vi "FV_Parameter.vi"(8 "error in (no error)":errorcluster, 11 "Ref in":T3={"MS SQL Connection"=refnum, "UDL File"=path "", "Time"="", "DCODE"="", "WIP+1"=0, "MC No?"=0, "POKAYOKE?"=FALSE, "Expected Result"="", "Result [Status]"="", "Clock"=0.0, "RFID"="", "WIP Queue"=refnum, "TS Parameter"={"ProfitCenterCode"="", "LineCode"="", "WorkOrderNumber"="", "Model"="", "Model_with_Prefix"="", "VendorCode"="", "SetParameterDateCode"="", "PokaYoke"=0, "Target"=1, "Live_DateCode"="", "CustomerPartNumber"="", "Hand"="", "sBarcode"=FALSE, "FCA"=0, "Ent_Stamp"=timestamp(0 s since 1904-01-01), "STS_CD"=0.0}, "Data_Queue"=[], "RFID Serial No."=""} {"TS Parameter"."FCA" format="%01d"; "TS Parameter"."Target" min=1 max=100000; "TS Parameter"."PokaYoke" min=0 max=1}) -> (0 "error out":errorcluster)   [LabVIEW 2020]
uses:
  Controls/TD SQL.ctl
  <vilib>/addons/database/Connection.llb/Conn ObjectReference.ctl
  Controls/WIP_State.ctl
  Controls/TS_Parameter.ctl
  Controls/FV_Operator.ctl
  <vilib>/Utility/miscctls.llb/LVPointTypeDef.ctl
  <vilib>/Utility/miscctls.llb/LVRowAndColumnUnsignedTypeDef.ctl
  <userlib>/_OpenG.lib/array/array.llb/Delete Elements from 1D Array (String)__ogtk.vi
  <vilib>/addons/database/NI_Database_API.lvlib
panel:
  in  "Exit":bool
  in  "Save wip":bool
  out "size(s)":i32
  in  "Add":bool
  in  "Remove":bool
  in  "Checking Tags":i32(listbox)
  in  "Avaliable Tags":i32(listbox)
  in  "FV_Check":T2 {"Tags" items=["PROFITCENTRE", "DTS_SCAN", "DTS_PASS", "DCODE", "SERIAL_NO", "BLEED_PORT_CNTY", "INLET_PORT_CNTY", "BLEED_TEST_TIME", "CLEANING_VAC", "CT", "STATUS", "FCS", "FCA", "ROUTING", "MODELNO", "WORKORDER", "CELLNO", "PROFITCENTRE", "MACHINECODE", "OPERATIONCODE", "RESERVED_1", "RESERVED_2", "RESERVED_3", "RESERVED_4", "RESERVED_5"]}
  out "Tags":string[](array[string])
  in  "Machine No":u16(ring) items=["OP20A", "OP20A", "OP20A", "OP20A"]
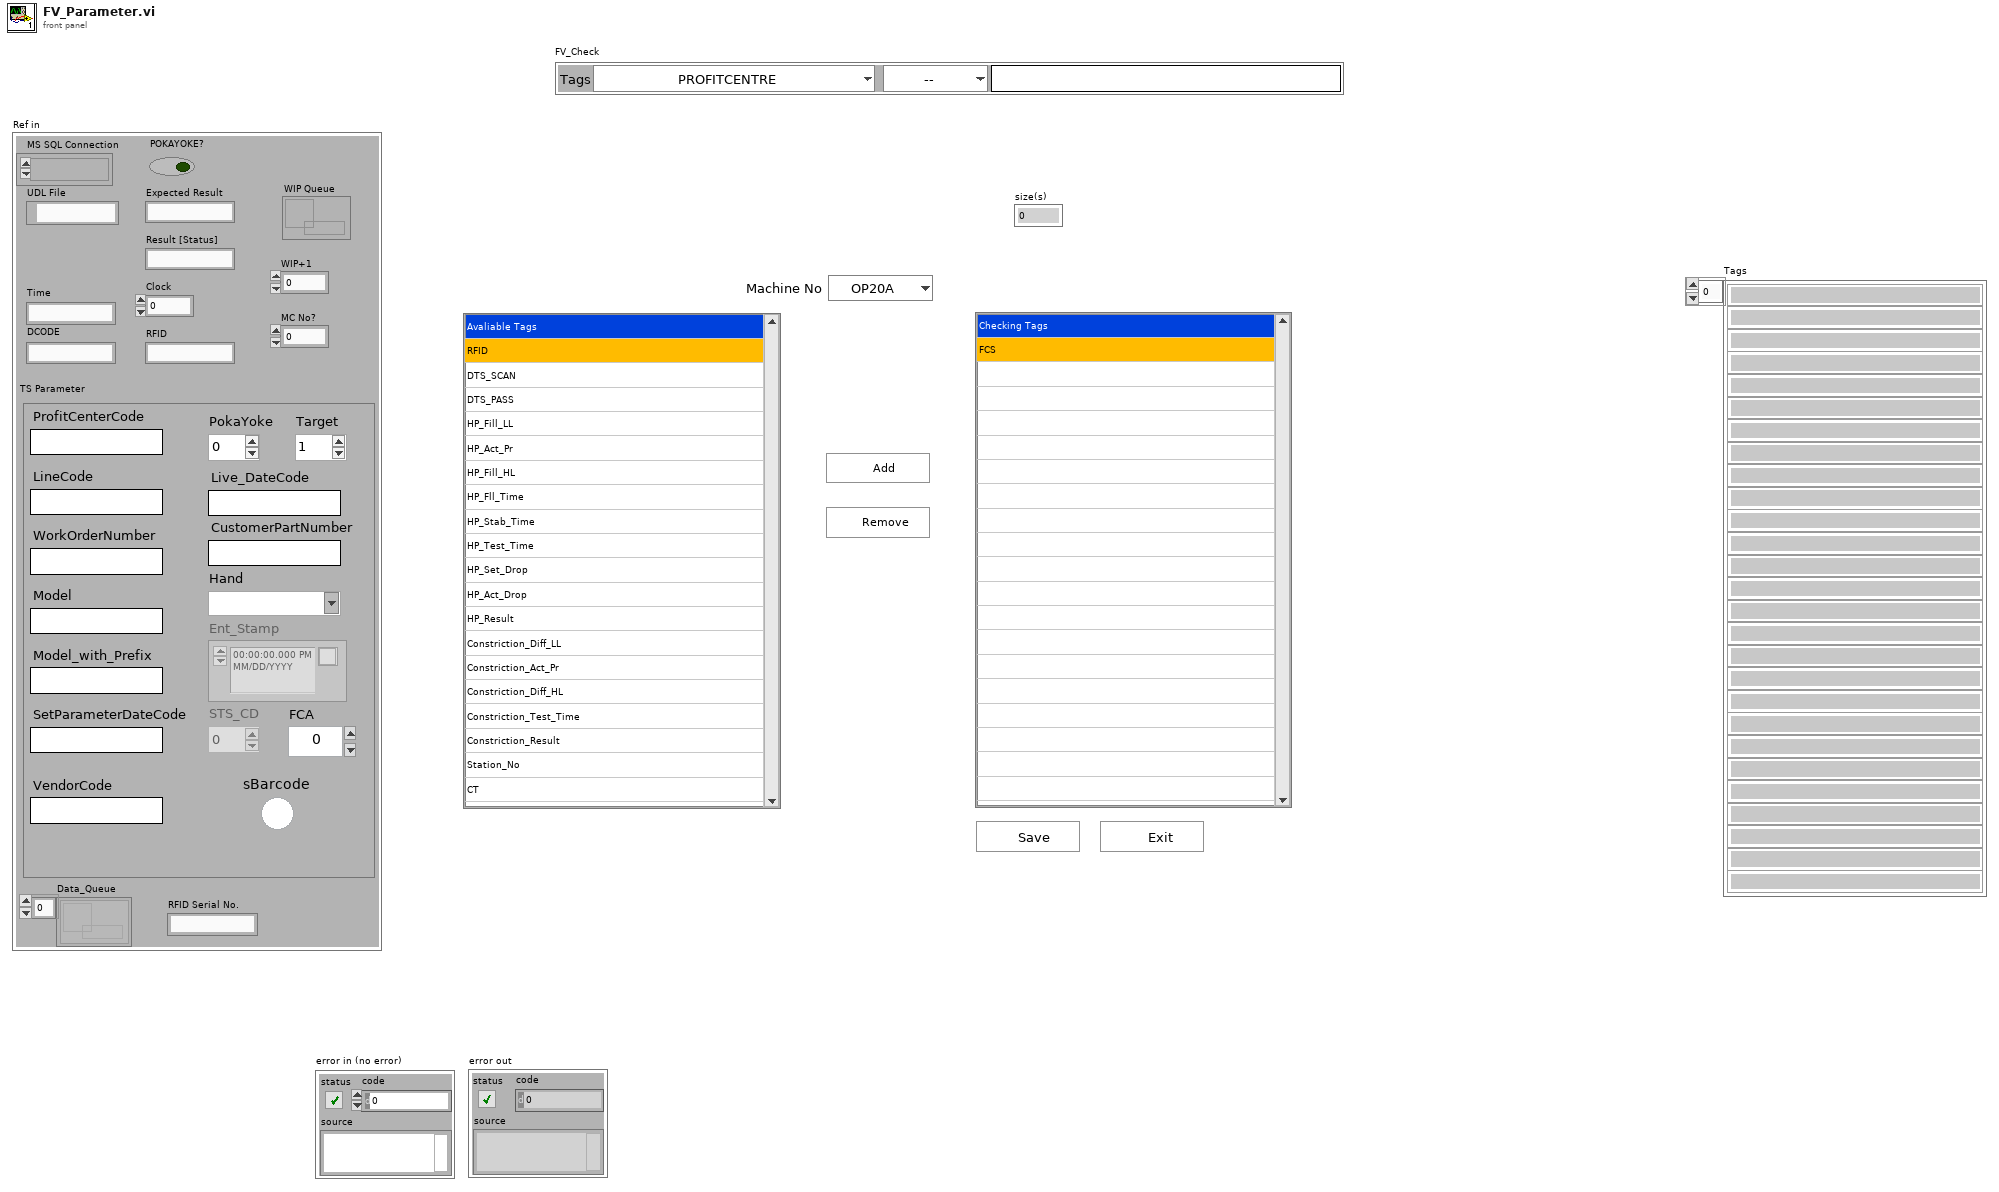
[diagram p1: front panel]
types:
  T1 = typedef "FV_Operator.ctl" = enum16{"--", "<", ">", "=", "Limits"}
  T2 = cluster{"Tags":u16, "Operator":T1, "Field":string}
  T3 = typedef "TD SQL.ctl" = cluster{"MS SQL Connection":T4, "UDL File":path, "Time":string, "DCODE":string, "WIP+1":i64, "MC No?":i32, "POKAYOKE?":bool, "Expected Result":string, "Result [Status]":string, "Clock":dbl, "RFID":string, "WIP Queue":refnum<queue>, "TS Parameter":T5, "Data_Queue":refnum<queue>[], "RFID Serial No.":string}
  T4 = typedef "NI_Database_API.lvlib/Conn ObjectReference.ctl" = refnum<k1>
  T5 = typedef "TS_Parameter.ctl" = cluster{"ProfitCenterCode":string, "LineCode":string, "WorkOrderNumber":string, "Model":string, "Model_with_Prefix":string, "VendorCode":string, "SetParameterDateCode":string, "PokaYoke":i32, "Target":i32, "Live_DateCode":string, "CustomerPartNumber":string, "Hand":string, "sBarcode":bool, "FCA":i32, "Ent_Stamp":timestamp, "STS_CD":dbl}
  T6 = typedef "LVPointTypeDef.ctl" = cluster{"Horizontal":i16, "Vertical":i16}
  T7 = enum8{"Enabled", "Disabled", "Disabled and Grayed Out"}
  T8 = typedef "LVRowAndColumnUnsignedTypeDef.ctl" = cluster{"Row":u32, "Column":u32}
  T9 = cluster{"data name":string, "drag data":variant}[]
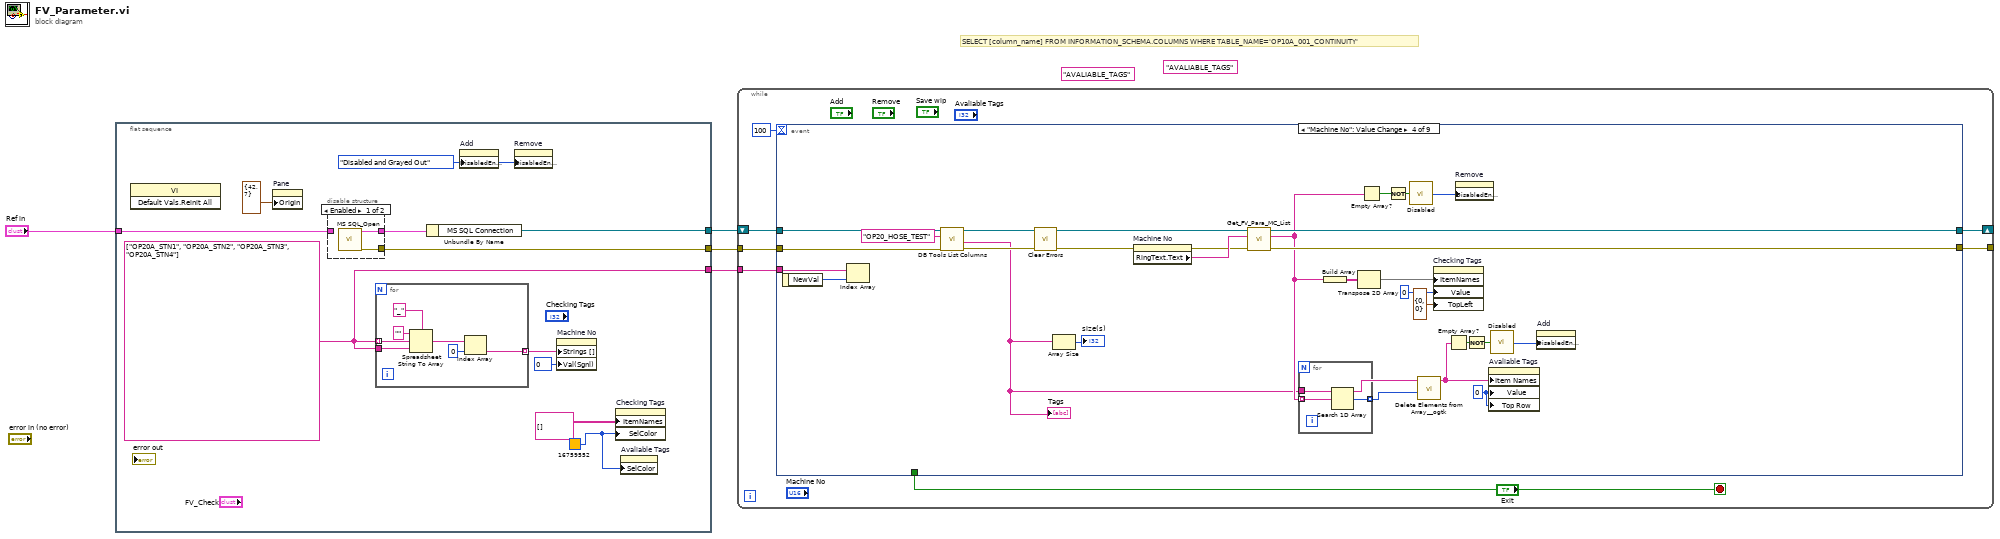
[diagram p0: block diagram]
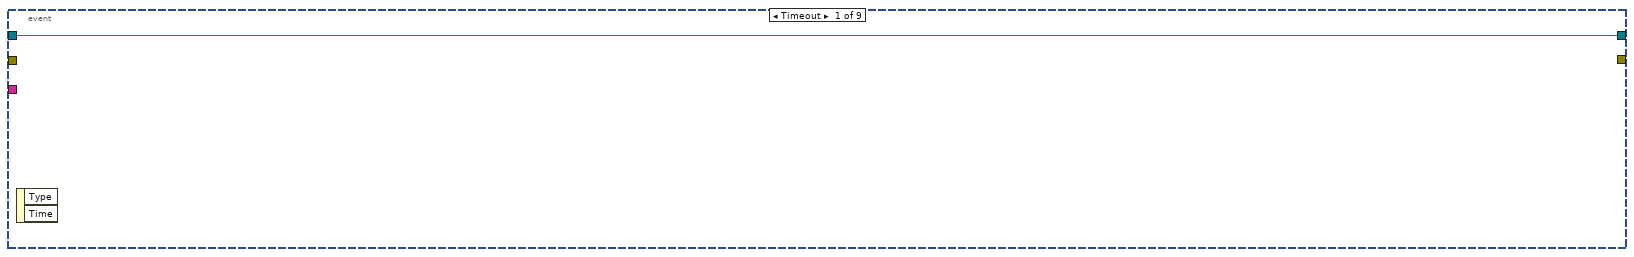
[diagram p3: hidden frame]
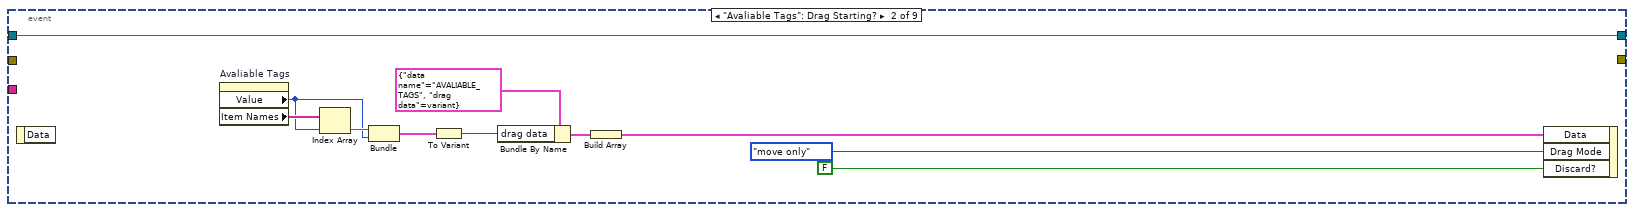
[diagram p4: hidden frame]
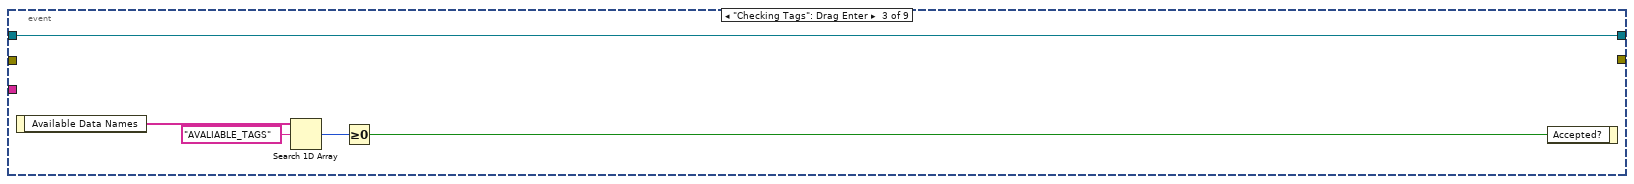
[diagram p5: hidden frame]
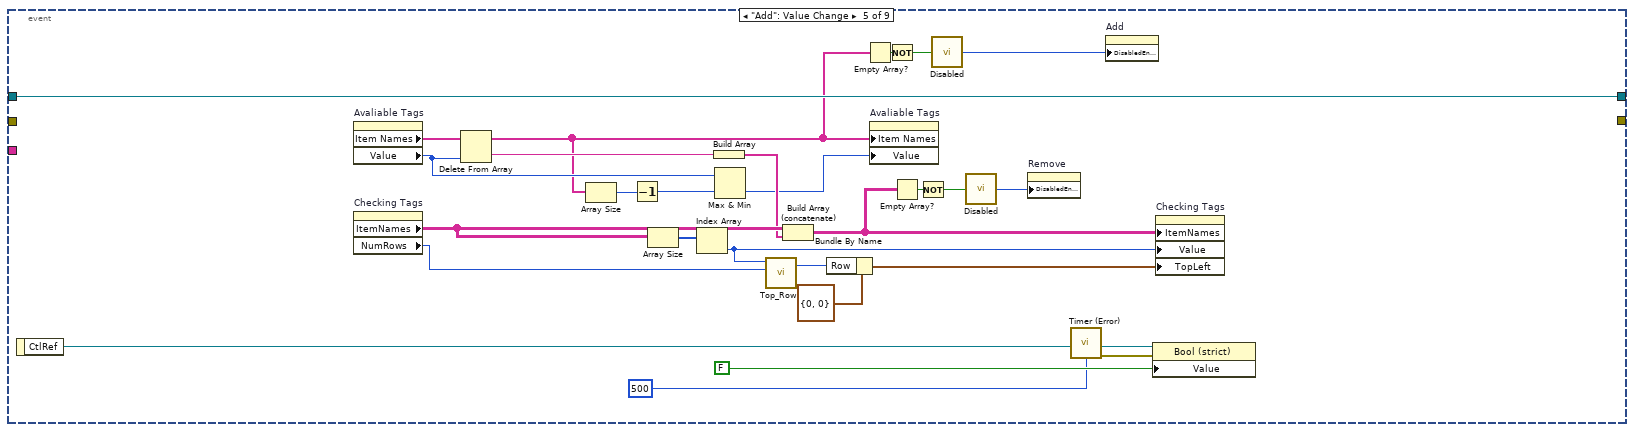
[diagram p6: hidden frame]
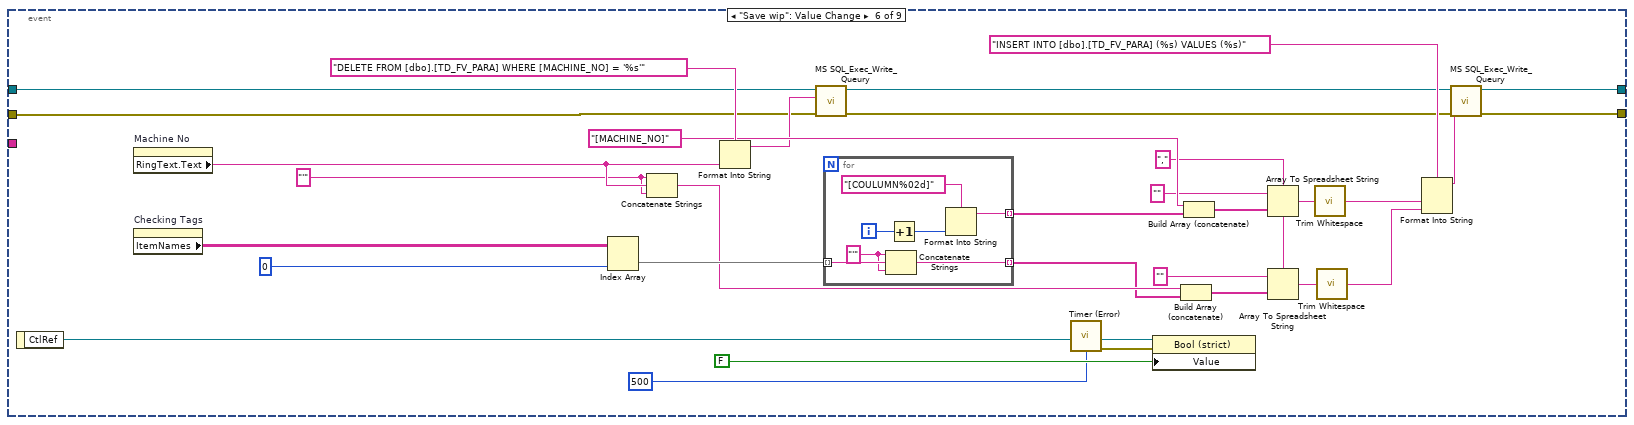
[diagram p7: hidden frame]
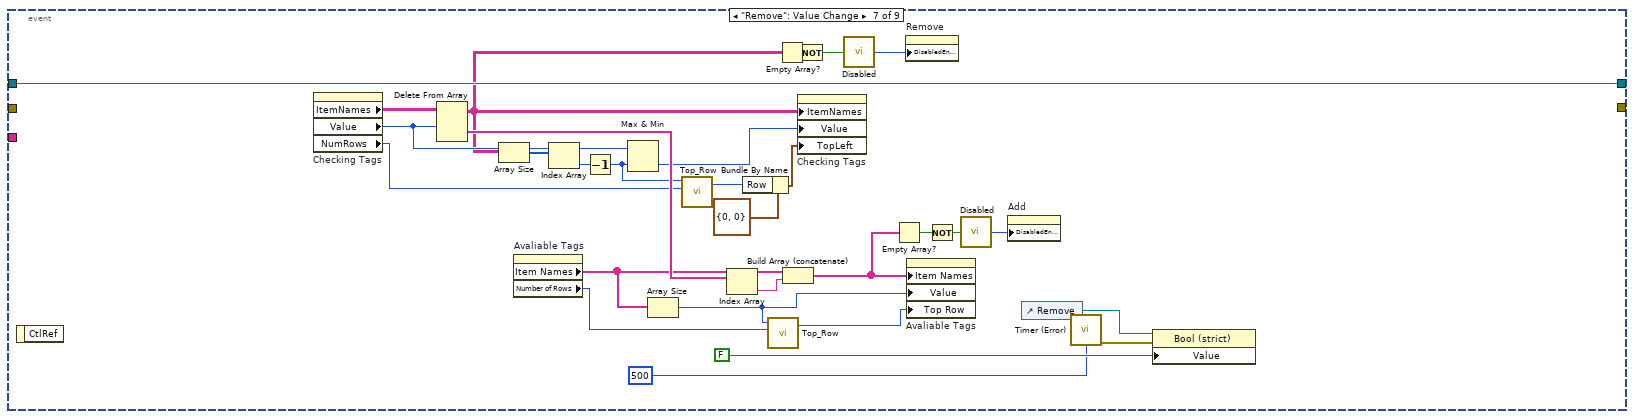
[diagram p8: hidden frame]
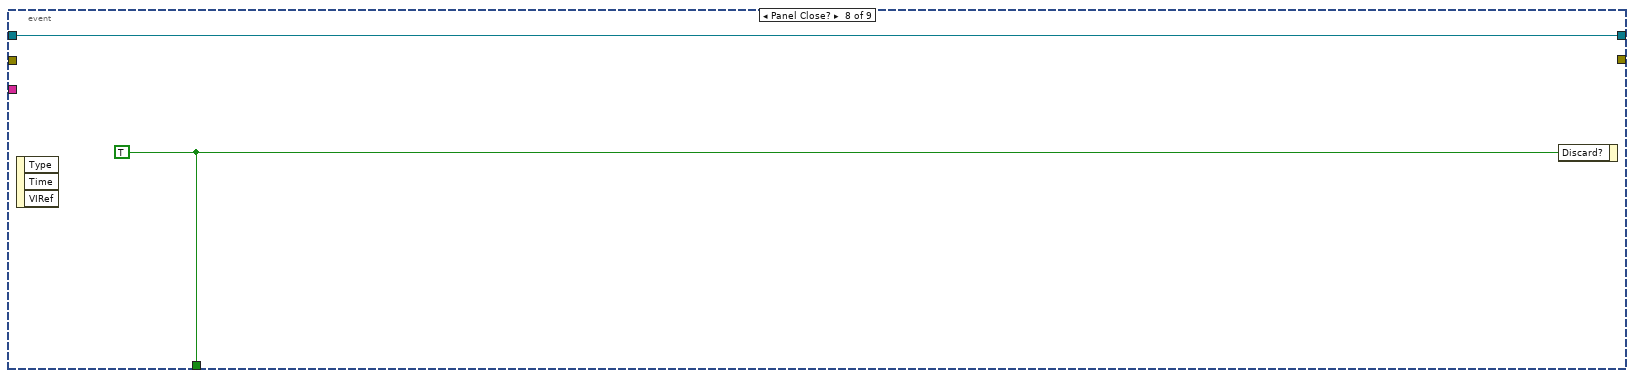
[diagram p9: hidden frame]
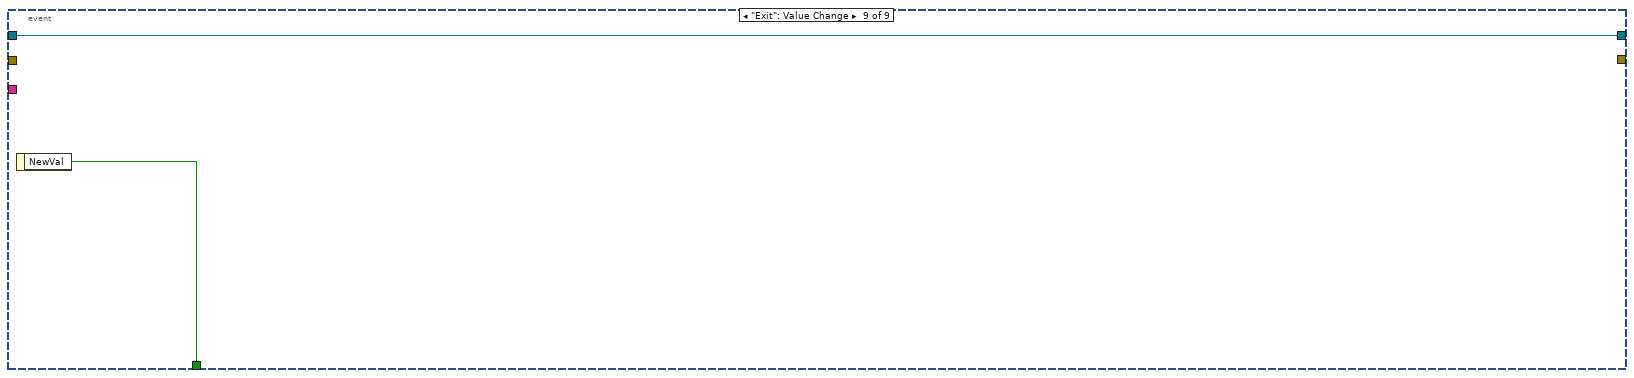
[diagram p10: hidden frame]
diagram:
  (unwired) "AVALIABLE_TAGS" ("data name")
  (unwired) "AVALIABLE_TAGS" ("data name")
  # "SELECT [column_name] FROM INFORMATION_SCHEMA.COLUMNS WHERE TABLE_NAME='OP10A_001_CONTINUITY'"
  n1 = flat-sequence {
    tunnel: "Ref in" -> [w14]
    tunnel: [w11] -> w1
    tunnel: [w10] -> w3
    tunnel: [w9] -> w2
    frame #0 {
      w6 = T7."Disabled and Grayed Out" ("Disabled")
      w7 = u32 16759552 ("Selection Color")
      w12 = u16 0 items=[""] ("Machine No")
      w10 = string[] ["OP20A_STN1", "OP20A_STN2", "OP20A_STN3", "OP20A_STN4"] ("tables 2")
      n2 = invoke class="VI" method="Default Vals.Reinit All"() -> ()  [unwired: 3 in, 3 out]
      n3 = property on="Pane" class="Pane"("Origin"=T6 {"Horizontal"=42, "Vertical"=7}) -> ()  [unwired: 2 in, 2 out]
      n4 = disable-structure shown="Enabled" {
        disable-tunnel: [w24 w25] -> w15
        disable-tunnel: w14 -> [_ w25]
        disable-tunnel: [w23 _] -> w9
        frame Enabled {
          n5 = call "MS SQL_Open.vi"() -> ("error out"=w23:errorcluster, "Ref Out"=w24:T3)  [unwired: 9 in, 1 out]
        }
        frame Disabled {
        }
      }
      n6 = for {
        tunnel: w10 -> [w18] mode=indexing
        tunnel: w10 -> [w17]
        tunnel: [w16] -> w13 mode=indexing
        n7 = Spreadsheet String To Array(delimiter (Tab)="_", format string="", spreadsheet string=w18, array type (2D Dbl)=w17) -> (array=w20:string[])
        n8 = Index Array(array=w20, index=0) -> (element=w16:string)
      }
      n9 = Unbundle By Name(w15) -> ("MS SQL Connection"=w11:T4)
      n10 = property on="Add" class="Bool (strict)"("DisabledEnum"=w6) -> ()  [unwired: 2 in, 2 out]
      n11 = property on="Remove" class="Bool (strict)"("DisabledEnum"=w6) -> ()  [unwired: 2 in, 2 out]
      n12 = property on="Machine No" class="Ring (strict)"("Strings []"=w13, "Val(Sgnl)"=w12) -> ()  [unwired: 2 in, 2 out]
      n13 = property on="Checking Tags" class="MCListbox (strict)"("ItemNames"=string[][] [] ("Item Names"), "SelColor"=w7) -> ()  [unwired: 2 in, 2 out]
      n14 = property on="Avaliable Tags" class="LstBox (strict)"("SelColor"=w7) -> ()  [unwired: 2 in, 2 out]
    }
  }
  n15 = while {
    tunnel: w3 -> [w31]
    tunnel: w2 -> [w30]
    tunnel: [w29] -> _
    shift-right: [w28] -> _
    shift-left: w1 -> [w27]
    stop <- w32 stop-if-true
    n16 = event shown="[3] \"Machine No\": Value Change" {
      selector: _ -> [_ _ _ _ _ _ _ _ _]
      dyn-events: _ -> [_ _ _ _ _ _ _ _ _]
      timeout: 100 -> [_ _ _ _ _ _ _ _ _]
      tunnel: [_ _ _ _ _ _ _ w177 w178] -> w32
      tunnel: w27 -> [w33 w44 w49 w66 w99 w115 w170 w176 w179]
      tunnel: w31 -> [_ _ _ w65 _ _ _ _ _]
      tunnel: w30 -> [_ _ _ w76 _ w113 _ _ _]
      tunnel: [_ _ _ w68 _ w109 _ _ _] -> w29
      tunnel: [w33 w44 w49 w69 w99 w108 w170 w176 w179] -> w28
      event Timeout {
        n17 = event-data() -> ()  [unwired: 1 in, 2 out]
      }
      event "Avaliable Tags": Drag Starting? {
        n18 = event-data() -> ()  [unwired: 1 in, 1 out]
        n19 = property on="Avaliable Tags" class="LstBox (strict)"() -> ("Value"=w39:i32, "Item Names"=w41:string[])  [unwired: 2 in, 2 out]
        n20 = Index Array(array=w41, index=w39) -> (element=w40:string)
        n21 = Bundle(w40, "Value"=w39) -> (w37:cluster{string, "Value":i32})  [unwired: 1 in]
        n22 = To Variant(anything=w37) -> (Variant=w34:variant)
        n23 = Bundle By Name(cluster=cluster{"data name":string, "drag data":variant} {"data name"="AVALIABLE_TAGS", "drag data"=variant}, "drag data"=w34) -> (w36:cluster{"data name":string, "drag data":variant})
        n24 = Build Array(w36) -> (w35:T9)
        n25 = event-data("Data"=w35, "Drag Mode"=enum32{"copy or move", "copy only", "move only"}."move only", "Discard?"=FALSE) -> ()  [unwired: 1 in, 1 out]
      }
      event "Checking Tags": Drag Enter {
        n26 = event-data() -> ("Available Data Names"=w47:string[])  [unwired: 1 in]
        n27 = Search 1D Array(1D array=w47, element="AVALIABLE_TAGS") -> (index of element=w48:i32)  [unwired: 1 in]
        n28 = Greater Or Equal To 0?(x=w48) -> (x >= 0?=w45:bool)
        n29 = event-data("Accepted?"=w45) -> ()  [unwired: 1 in, 1 out]
      }
      event "Machine No": Value Change {
        w56 = 0 ("Avaliable Tags")
        n30 = event-data() -> ("NewVal"=w77:u16)  [unwired: 1 in]
        n31 = Index Array(array=w65, index=w77) -> ()  [unwired: 1 out]
        n32 = call <vilib>:"DB Tools List Columns.vi"("error in (no error)"=w76, "table"="OP20_HOSE_TEST", "connection reference"=w66) -> ("error out"=w74:errorcluster, "columns"=w53:string[], "connection reference out"=w67:T4)  [unwired: 1 in, 1 out]
        "Tags" <- w53
        n33 = call <vilib>:"Clear Errors.vi"("error in (no error)"=w74) -> ("error out"=w52:errorcluster)  [unwired: 5 in, 1 out]
        n34 = Array Size(array=w53) -> (size(s)=→"size(s)":i32)
        n35 = property on="Machine No" class="Ring (strict)"(error in=w52) -> (error out=w51:errorcluster, "RingText.Text"=w72:string)  [unwired: 1 in, 1 out]
        n36 = call "Get_FV_Para_MC_List.vi"("error in (no error)"=w51, "Machine No."=w72, "Refnum in"=w67) -> ("error out"=w68:errorcluster, "Column"=w57:string[], "Refnum out"=w69:T4)  [unwired: 3 in, 3 out]
        n37 = for {
          tunnel: w53 -> [w80]
          tunnel: w57 -> [w79] mode=indexing
          tunnel: [w78] -> w70 mode=indexing
          n38 = Search 1D Array(1D array=w80, element=w79) -> (index of element=w78:i32)  [unwired: 1 in]
        }
        n39 = Build Array(w57) -> (w73:string[][])
        n40 = Transpose 2D Array(2D array=w73) -> (transposed array=w71:string[][])
        n41 = Empty Array?(array=w57) -> (empty?=w64:bool)
        n42 = Not(x=w64) -> (.not. x?=w59:bool)
        n43 = call <userlib>:"Disabled.vi"("Enable?"=w59) -> ("Disabled"=w63:T7)  [unwired: 14 in]
        n44 = call-poly <userlib>:"Delete Elements from Array__ogtk.vi"("indices"=w70, "array"=w53) -> ("array w/ subset deleted"=w60:string[])  [unwired: 8 in, 1 out]
        n45 = property on="Checking Tags" class="MCListbox (strict)"("ItemNames"=w71, "Value"=0 ("Checking Tags"), "TopLeft"=T8 {"Row"=0, "Column"=0} ("Top Left Visible Cell")) -> ()  [unwired: 2 in, 2 out]
        n46 = Empty Array?(array=w60) -> (empty?=w62:bool)
        n47 = property on="Remove" class="Bool (strict)"("DisabledEnum"=w63) -> ()  [unwired: 2 in, 2 out]
        n48 = Not(x=w62) -> (.not. x?=w58:bool)
        n49 = property on="Avaliable Tags" class="LstBox (strict)"("Item Names"=w60, "Value"=w56, "Top Row"=w56) -> ()  [unwired: 2 in, 2 out]
        n50 = call <userlib>:"Disabled.vi"("Enable?"=w58) -> ("Disabled"=w61:T7)  [unwired: 14 in]
        n51 = property on="Add" class="Bool (strict)"("DisabledEnum"=w61) -> ()  [unwired: 2 in, 2 out]
      }
      event "Add": Value Change {
        n52 = event-data() -> ("CtlRef"=w103:refnum<vi>)  [unwired: 1 in]
        n53 = property on="Avaliable Tags" class="LstBox (strict)"() -> ("Item Names"=w107:string[], "Value"=w97:i32)  [unwired: 2 in, 2 out]
        n54 = property on="Checking Tags" class="MCListbox (strict)"() -> ("ItemNames"=w105:string[][], "NumRows"=w82:u32)  [unwired: 2 in, 2 out]
        n55 = Delete From Array(array=w107, index=w97) -> (deleted portion=w106:string, array with subset deleted=w93:string[])  [unwired: 1 in]
        n56 = Array Size(array=w93) -> (size(s)=w96:i32)
        n57 = Decrement(x=w96) -> (x-1=w95:i32)
        n58 = Array Size(array=w105) -> (size(s)=w104:i32[])
        n59 = Index Array(array=w104) -> (element=w83:i32)  [unwired: 1 in]
        n60 = Build Array(w106) -> (w98:string[])
        n61 = Max & Min(x=w97, y=w95) -> (min(x,y)=w94:i32)  [unwired: 1 out]
        n62 = call "Top_Row.vi"("NumRows"=w82, "Step In"=w83) -> ("Step Out"=w81:i32)  [unwired: 3 in]
        n63 = Build Array (concatenate)(w105, w98) -> (w89:string[][])
        n64 = Bundle By Name(cluster=T8 {"Row"=0, "Column"=0} ("Top Left Visible Cell"), "Row"=w81) -> (w84:T8)
        n65 = Empty Array?(array=w93) -> (empty?=w92:bool)
        n66 = property on="Avaliable Tags" class="LstBox (strict)"("Item Names"=w93, "Value"=w94) -> ()  [unwired: 2 in, 2 out]
        n67 = Not(x=w92) -> (.not. x?=w87:bool)
        n68 = Empty Array?(array=w89) -> (empty?=w90:bool)
        n69 = Not(x=w90) -> (.not. x?=w86:bool)
        n70 = call <userlib>:"Disabled.vi"("Enable?"=w87) -> ("Disabled"=w91:T7)  [unwired: 14 in]
        n71 = call <userlib>:"Disabled.vi"("Enable?"=w86) -> ("Disabled"=w88:T7)  [unwired: 14 in]
        n72 = property on="Remove" class="Bool (strict)"("DisabledEnum"=w88) -> ()  [unwired: 2 in, 2 out]
        n73 = call <userlib>:"Timer (Error).vi"("milliseconds to wait"=u32 500) -> ("error out"=w100:errorcluster)  [unwired: 14 in]
        n74 = property on="Add" class="Bool (strict)"("DisabledEnum"=w91) -> ()  [unwired: 2 in, 2 out]
        n75 = property class="Bool (strict)"(reference=w103, error in=w100, "Value"=FALSE) -> ()  [unwired: 2 out]
        n76 = property on="Checking Tags" class="MCListbox (strict)"("ItemNames"=w89, "Value"=w83, "TopLeft"=w84) -> ()  [unwired: 2 in, 2 out]
      }
      event "Save wip": Value Change {
        w117 = "'" ("string")
        w121 = "," ("delimiter (Tab)")
        n77 = event-data() -> ("CtlRef"=w139:refnum<vi>)  [unwired: 1 in]
        n78 = property on="Machine No" class="Ring (strict)"() -> ("RingText.Text"=w132:string)  [unwired: 2 in, 2 out]
        n79 = property on="Checking Tags" class="MCListbox (strict)"() -> ("ItemNames"=w134:string[][])  [unwired: 2 in, 2 out]
        n80 = Index Array(array=w134, index (col)=0 ("disabled index (col)")) -> (element=w131:string[])  [unwired: 1 in]
        n81 = Concatenate Strings(w117, w132, w117) -> (w118:string)
        n82 = Format Into String(format string="DELETE FROM [dbo].[TD_FV_PARA] WHERE [MACHINE_NO] = '%s'" ("SQL query"), w132) -> (resulting string=w114:string)  [unwired: 2 in, 1 out]
        n83 = call "MS SQL_Exec_Write_Queury.vi"("error in (no error)"=w113, "Query"=w114, "Refnum in"=w115) -> ("error out"=w111:errorcluster, "Refnum out"=w112:T4)  [unwired: 7 in]
        n84 = for {
          tunnel: w131 -> [w142] mode=indexing
          tunnel: [w143] -> w130 mode=indexing
          tunnel: [w140] -> w116 mode=indexing
          i -> [w146]
          w141 = "'" ("string")
          n85 = Concatenate Strings(w141, w142, w141) -> (w140:string)
          n86 = Increment(x=w146) -> (x+1=w144:i32)
          n87 = Format Into String(format string="[COULUMN%02d]", w144) -> (resulting string=w143:string)  [unwired: 2 in, 1 out]
        }
        n88 = call <userlib>:"Timer (Error).vi"("milliseconds to wait"=u32 500) -> ("error out"=w136:errorcluster)  [unwired: 14 in]
        n89 = property class="Bool (strict)"(reference=w139, error in=w136, "Value"=FALSE) -> ()  [unwired: 2 out]
        n90 = Build Array (concatenate)(w118, w116) -> (w125:string[])
        n91 = Build Array (concatenate)("[MACHINE_NO]" ("format string"), w130) -> (w129:string[])
        n92 = Array To Spreadsheet String(delimiter (Tab)=w121, array=w129, 3:"" ("format string")) -> (spreadsheet string=w123:string)
        n93 = Array To Spreadsheet String(delimiter (Tab)=w121, array=w125, 3:"" ("format string")) -> (spreadsheet string=w122:string)
        n94 = call <vilib>:"Trim Whitespace.vi"("string"=w123) -> ("trimmed string"=w120:string)  [unwired: 1 in]
        n95 = call <vilib>:"Trim Whitespace.vi"("string"=w122) -> ("trimmed string"=w119:string)  [unwired: 1 in]
        n96 = Format Into String(format string="INSERT INTO [dbo].[TD_FV_PARA] (%s) VALUES (%s)" ("SQL query"), w120, w119) -> (resulting string=w110:string)  [unwired: 2 in, 1 out]
        n97 = call "MS SQL_Exec_Write_Queury.vi"("error in (no error)"=w111, "Query"=w110, "Refnum in"=w112) -> ("error out"=w109:errorcluster, "Refnum out"=w108:T4)  [unwired: 7 in]
      }
      event "Remove": Value Change {
        n98 = event-data() -> ()  [unwired: 1 in, 1 out]
        n99 = property on="Checking Tags" class="MCListbox (strict)"() -> ("ItemNames"=w159:string[][], "Value"=w157:i32, "NumRows"=w152:u32)  [unwired: 2 in, 2 out]
        n100 = Delete From Array(array=w159, index (row)=w157) -> (deleted portion=w175:string[], array with subset deleted=w155:string[][])  [unwired: 2 in]
        n101 = Array Size(array=w155) -> (size(s)=w160:i32[])
        n102 = property on="Avaliable Tags" class="LstBox (strict)"() -> ("Item Names"=w174:string[], "Number of Rows"=w149:u32)  [unwired: 2 in, 2 out]
        n103 = Index Array(array=w160) -> (element=w158:i32)  [unwired: 1 in]
        n104 = Decrement(x=w158) -> (x-1=w151:i32)
        n105 = Max & Min(x=w157, y=w151) -> (min(x,y)=w156:i32)  [unwired: 1 out]
        n106 = Array Size(array=w174) -> (size(s)=w148:i32)
        n107 = call "Top_Row.vi"("NumRows"=w152, "Step In"=w151) -> ("Step Out"=w153:i32)  [unwired: 3 in]
        n108 = Index Array(array=w175) -> (element=w169:string)  [unwired: 1 in]
        n109 = Bundle By Name(cluster=T8 {"Row"=0, "Column"=0} ("Top Left Visible Cell"), "Row"=w153) -> (w150:T8)
        n110 = call "Top_Row.vi"("NumRows"=w149, "Step In"=w148) -> ("Step Out"=w161:i32)  [unwired: 3 in]
        n111 = Empty Array?(array=w155) -> (empty?=w165:bool)
        n112 = Build Array (concatenate)(w174, w169) -> (w166:string[])
        n113 = Not(x=w165) -> (.not. x?=w163:bool)
        n114 = property on="Checking Tags" class="MCListbox (strict)"("ItemNames"=w155, "Value"=w156, "TopLeft"=w150) -> ()  [unwired: 2 in, 2 out]
        n115 = call <userlib>:"Disabled.vi"("Enable?"=w163) -> ("Disabled"=w164:T7)  [unwired: 14 in]
        n116 = Empty Array?(array=w166) -> (empty?=w168:bool)
        n117 = property on="Remove" class="Bool (strict)"("DisabledEnum"=w164) -> ()  [unwired: 2 in, 2 out]
        n118 = property on="Avaliable Tags" class="LstBox (strict)"("Item Names"=w166, "Value"=w148, "Top Row"=w161) -> ()  [unwired: 2 in, 2 out]
        n119 = Not(x=w168) -> (.not. x?=w162:bool)
        n120 = call <userlib>:"Disabled.vi"("Enable?"=w162) -> ("Disabled"=w167:T7)  [unwired: 14 in]
        n121 = property on="Add" class="Bool (strict)"("DisabledEnum"=w167) -> ()  [unwired: 2 in, 2 out]
        n122 = control-ref of="Remove"() -> (w147:refnum<vi>)
        n123 = call <userlib>:"Timer (Error).vi"("milliseconds to wait"=u32 500) -> ("error out"=w171:errorcluster)  [unwired: 14 in]
        n124 = property class="Bool (strict)"(reference=w147, error in=w171, "Value"=FALSE) -> ()  [unwired: 2 out]
      }
      event Panel Close? {
        w177 = TRUE ("Discard?")
        n125 = event-data() -> ()  [unwired: 1 in, 3 out]
        n126 = event-data("Discard?"=w177) -> ()  [unwired: 1 in, 1 out]
      }
      event "Exit": Value Change {
        n127 = event-data() -> ("NewVal"=w178:bool)  [unwired: 1 in]
      }
    }
  }
